vi "OneShotButton.vi"(10 "Boolean":bool) -> (2 "Boolean 2":bool)   [LabVIEW 2018]
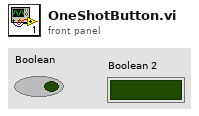
[diagram p1: front panel]
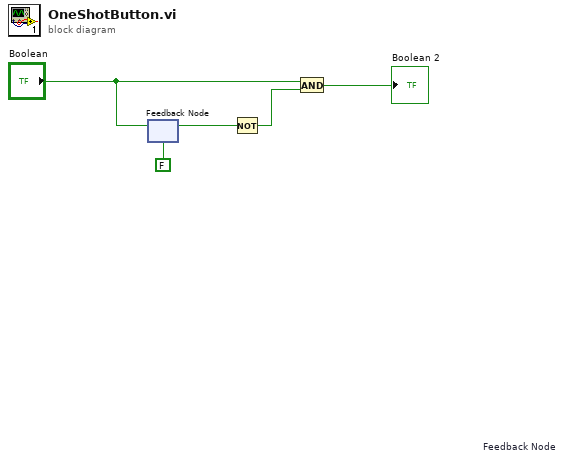
[diagram p0: block diagram]
diagram:
  n1 = feedback #1 "Feedback Node"(FALSE ("Button In")) -> (w5:bool)
  n2 = feedback-in #1("Boolean") -> ()
  n3 = Not(x=w5) -> (.not. x?=w4:bool)
  n4 = And(x="Boolean", y=w4) -> (x .and. y?=→"Boolean 2":bool)
